vi "LS330_TimedWriter.vi"(5 "Time Stamp":timestamp, 7 "Status In":cluster{T1, T1}, 8 "error in (no error)":errorcluster, 9 "Time Check In":timestamp, 10 "Interval":dbl, 11 "Byte Stream File in":refnum<file>) -> (0 "error out":errorcluster, 1 "Time Check Out":timestamp, 3 "Byte Stream File out":refnum<file>)   [LabVIEW 2021]
uses:
  LS330_Status_Bundle.ctl
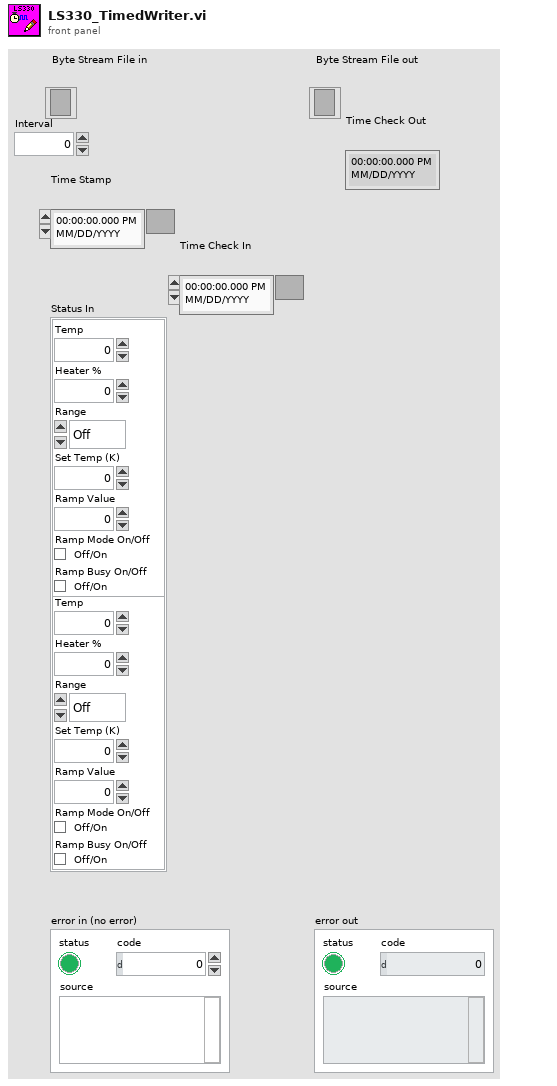
[diagram p1: front panel]
types:
  T1 = typedef "LS330_Status_Bundle.ctl" = cluster{"Temp":dbl, "Heater %":dbl, "Range":enum16{"Off", "Low", "Medium", "High"}, "Set Temp (K)":dbl, "Ramp Value":dbl, "Ramp Mode On/Off":bool, "Ramp Busy On/Off":bool}
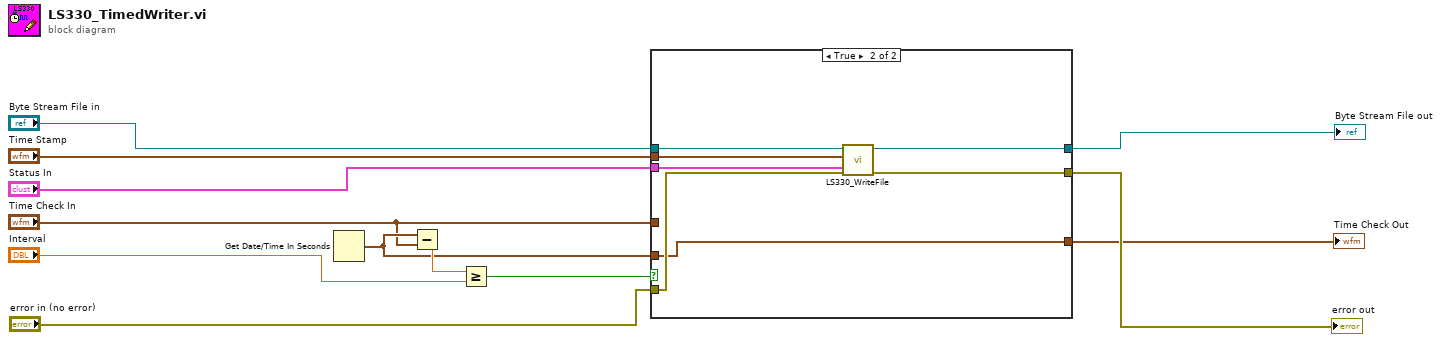
[diagram p0: block diagram]
diagram:
  n1 = Get Date/Time In Seconds() -> (seconds since 1Jan1904=w3:timestamp)
  n2 = Subtract(x=w3, y="Time Check In") -> (x-y=w5:dbl)
  n3 = Greater Or Equal?(x=w5, y="Interval") -> (x >= y?=w4:bool)
  n4 = case shown="True" w4 {
    tunnel: "Status In" -> [_ w22]
    tunnel: "Time Stamp" -> [_ w21]
    tunnel: [w14 w20] -> w10
    tunnel: [w15 w19] -> w9
    tunnel: "Byte Stream File in" -> [w15 w18]
    tunnel: "error in (no error)" -> [w14 w17]
    tunnel: w3 -> [_ w16]
    tunnel: "Time Check In" -> [w13 _]
    tunnel: [w13 w16] -> w1
    frame False {
    }
    frame True {
      n5 = call "LS330_WriteFile.vi"("error in"=w17, "Status IN"=w22, "current time"=w21, "File Ref in"=w18) -> ("error out"=w20:errorcluster, "refnum out"=w19:refnum<file>)  [unwired: 6 in]
    }
  }
  "error out" <- w10
  "Byte Stream File out" <- w9
  "Time Check Out" <- w1
